vi "XNET Create Session (Frame Output Single-point).vi"(5 "frame list":refnum<k21>[](array[refnum]), 9 "interface":refnum<k21>, 11 "error in (no error)":errorcluster) -> (4 "session out":refnum<k21>, 15 "error out":errorcluster)   [LabVIEW 2018]
doc: "Creates an XNET session at run time for the Frame Output Single-Point mode."
uses:
  XNET Mode.ctl
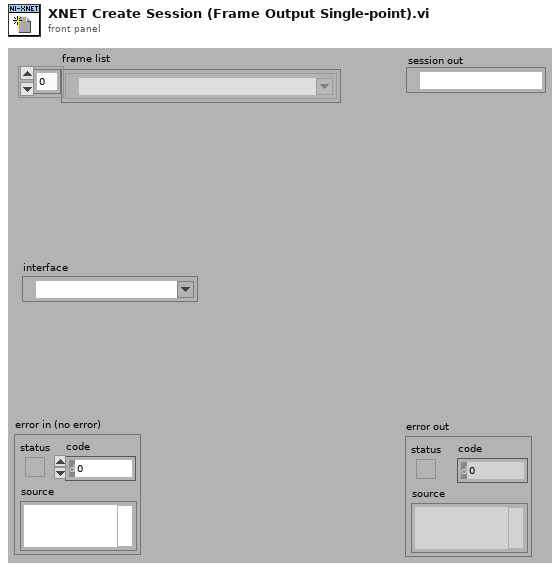
[diagram p1: front panel]
types:
  T1 = typedef "XNET Mode.ctl" = u32
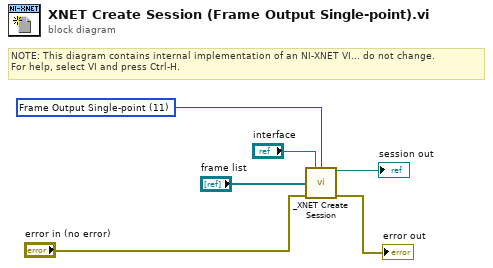
[diagram p0: block diagram]
diagram:
  w2 = T1 11 items=["Signal Input Single-point", "Signal Input Waveform", "Signal Input XY", "Signal Output Single-point", "Signal Output Waveform", "Signal Output XY", "Frame Input Stream", "Frame Input Queued", "Frame Input Single-point", "Frame Output Stream", "Frame Output Queued", "Frame Output Single-point"] ("mode")
  # "NOTE: This diagram contains internal implementation of an NI-XNET VI... do not change. \nFor help, select VI and press Ctrl-H."
  n1 = call "_XNET Create Session.vi"("interface"="interface", "mode"=w2, "signal/frame list (empty)"="frame list", "error in (no error)"="error in (no error)") -> ("session out"=→"session out":refnum<k21>, "error out"=→"error out":errorcluster)  [unwired: 10 out]
